vi "Elevator Teleop.vi"(8 "Disabled":bool, 11 "Cluster":T1) -> ()   [LabVIEW 2018]
uses:
  Support Code/Joystick Vals.ctl
  Implementation/Infrastructure/Positions.ctl
  Framework/Robot Global Data.vi
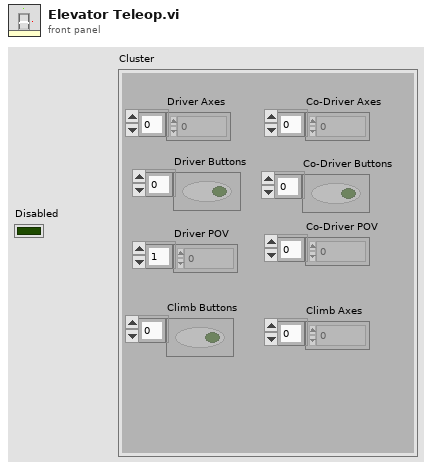
[diagram p1: front panel]
types:
  T1 = typedef "Joystick Vals.ctl" = cluster{"Driver Axes":dbl[], "Co-Driver Axes":dbl[], "Driver Buttons":bool[], "Co-Driver Buttons":bool[], "Driver POV":i16[], "Co-Driver POV":i16[], "Climb Buttons":bool[], "Climb Axes":dbl[]}
  T2 = typedef "Positions.ctl" = enum16{"MANUAL", "Bottom Pannel", "Bottom Cargo", "Feeder Station", "Cargo Ship Cargo", "Middle Pannel", "Middle Cargo", "Top Pannel", "Top Cargo"}
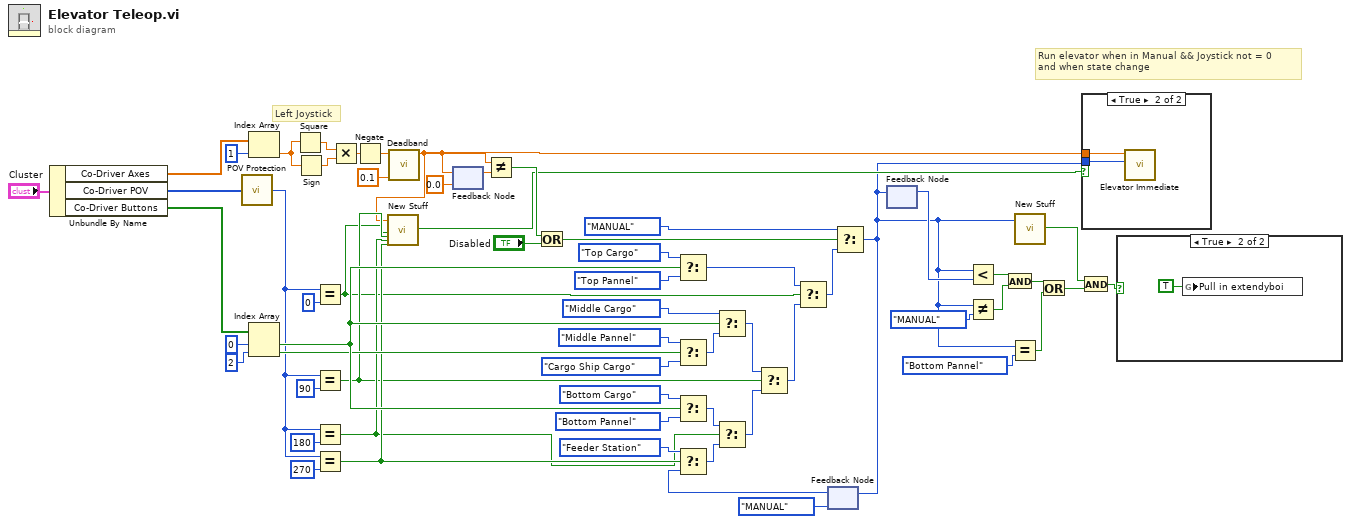
[diagram p0: block diagram]
diagram:
  # "Run elevator when in Manual && Joystick not = 0\nand when state change"
  # "Left Joystick"
  n1 = Unbundle By Name("Cluster") -> ("Co-Driver Axes"=w60:dbl[], "Co-Driver POV"=w23:i16[], "Co-Driver Buttons"=w53:bool[])
  n2 = call "POV Protection.vi"("Array"=w23) -> ("s? t:f"=w18:i32)
  n3 = Index Array(array=w60, index=1) -> (element=w34:dbl)
  n4 = Index Array(array=w53, index #1=0 ("index"), index #2=2 ("index")) -> (element #1=w39:bool, element #2=w22:bool)
  n5 = Square(x=w34) -> (x^2=w36:dbl)
  n6 = Sign(1:w34) -> (0:w35:dbl)
  n7 = Equal?(x=w18, y=i16 0) -> (x = y?=w8:bool)
  n8 = Equal?(x=w18, y=i16 90) -> (x = y?=w9:bool)
  n9 = Equal?(x=w18, y=i16 180) -> (x = y?=w10:bool)
  n10 = Equal?(x=w18, y=i16 270) -> (x = y?=w11:bool)
  n11 = Multiply(x=w36, y=w35) -> (x*y=w33:dbl)
  n12 = Negate(x=w33) -> (-x=w32:dbl)
  n13 = call "Deadband.vi"("Deadband"=0.1, "Input"=w32) -> ("f"=w6:dbl)  [unwired: 9 in]
  n14 = call "New Stuff.vi"("Variant 2"=w6, "Variant 16"=w8, "Variant 15"=w9, "Variant 8"=w10, "Variant 7"=w11) -> ("x != y?"=w7:bool)  [unwired: 22 in]
  n15 = feedback-in #1(w6) -> ()
  n16 = feedback #1(0.0 ("f")) -> (w38:dbl)
  n17 = Not Equal?(x=w6, y=w38) -> (x != y?=w26:bool)
  n18 = Or(x=w26, y="Disabled") -> (x .or. y?=w25:bool)
  n19 = Select(t=Positions."Top Cargo" ("Position"), s=w39, f=Positions."Top Pannel" ("Position")) -> (s? t:f=w41:T2)
  n20 = Select(t=Positions."Middle Pannel" ("Position"), s=w22, f=Positions."Cargo Ship Cargo" ("Position")) -> (s? t:f=w19:T2)
  n21 = Select(t=Positions."Bottom Cargo" ("Position"), s=w39, f=Positions."Bottom Pannel" ("Position")) -> (s? t:f=w47:T2)
  n22 = Select(t=Positions."Middle Cargo" ("Position"), s=w39, f=w19) -> (s? t:f=w44:T2)
  n23 = feedback #2(Positions."MANUAL" ("Position")) -> (w29:T2)
  n24 = Select(t=Positions."Feeder Station" ("Position"), s=w11, f=w29) -> (s? t:f=w28:T2)
  n25 = Select(t=w47, s=w10, f=w28) -> (s? t:f=w46:T2)
  n26 = Select(t=w44, s=w9, f=w46) -> (s? t:f=w40:T2)
  n27 = Select(t=w41, s=w8, f=w40) -> (s? t:f=w56:T2)
  n28 = Select(t=Positions."MANUAL" ("Position"), s=w25, f=w56) -> (s? t:f=w1:T2)
  n29 = feedback-in #2(w1) -> ()
  n30 = feedback-in #3(w1) -> ()
  n31 = feedback #3() -> (w17:T2)  [unwired: 1 in]
  n32 = Less?(x=w1, y=w17) -> (x < y?=w16:bool)
  n33 = Not Equal?(x=w1, y=Positions."MANUAL" ("Position")) -> (x != y?=w15:bool)
  n34 = And(x=w16, y=w15) -> (x .and. y?=w3:bool)
  n35 = Equal?(x=w1, y=Positions."Bottom Pannel" ("Position")) -> (x = y?=w13:bool)
  n36 = call "New Stuff.vi"("Variant 2"=w1) -> ("x != y?"=w2:bool)  [unwired: 26 in]
  n37 = Or(x=w3, y=w13) -> (x .or. y?=w5:bool)
  n38 = And(x=w2, y=w5) -> (x .and. y?=w4:bool)
  n39 = case shown="True" w7 {
    tunnel: w6 -> [_ w63]
    tunnel: w1 -> [_ w62]
    frame False {
    }
    frame True {
      n40 = call "Elevator Immediate.vi"("Position"=w62, "Setpoint"=w63) -> ()  [unwired: 9 in, 1 out]
    }
  }
  n41 = case shown="True" w4 {
    frame False {
    }
    frame True {
      n42 = global write "Robot Global Data.vi" "Pull in extendyboi"(TRUE ("Pull in extendyboi")) -> ()
    }
  }
